vi "EnqueueCommand.vi"(8 "error in (no error)":errorcluster, 10 "element":T1, 11 "ResultProcessor in":refnum<class "ResultProcessor.lvclass">) -> (0 "error out":errorcluster, 3 "ResultProcessor out":refnum<class "ResultProcessor.lvclass">)   [LabVIEW 2015, in "ResultProcessor.lvclass"]
uses:
  ResultProcessor.lvclass
  CommandQueueDataType.ctl
  Report Information/Report Information.lvclass
  Result/Result.lvclass
  ResultProcessor.lvclass/ResultProcessor.ctl
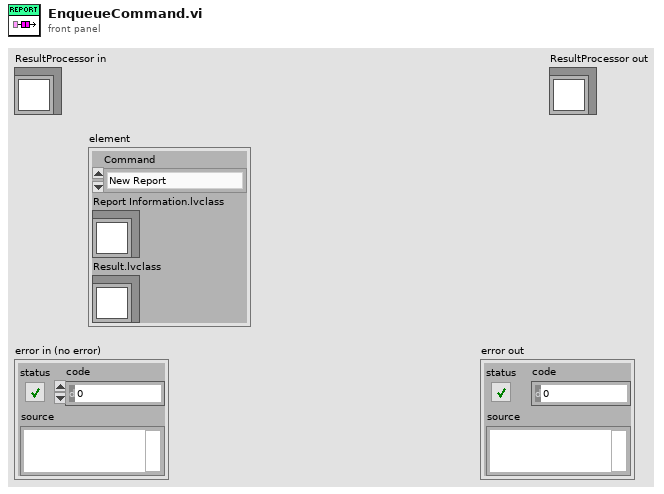
[diagram p1: front panel]
types:
  T1 = typedef "ResultProcessor.lvclass/CommandQueueDataType.ctl" = cluster{"Command":enum16{"New Report", "Add Result", "Publish Report", "Shutdown", "Add DUT Information", "Add Station Information", "Add Report Information", "Add Test Information"}, "Report Information.lvclass":refnum<class "Report Information.lvclass">, "Result.lvclass":refnum<class "Result.lvclass">}
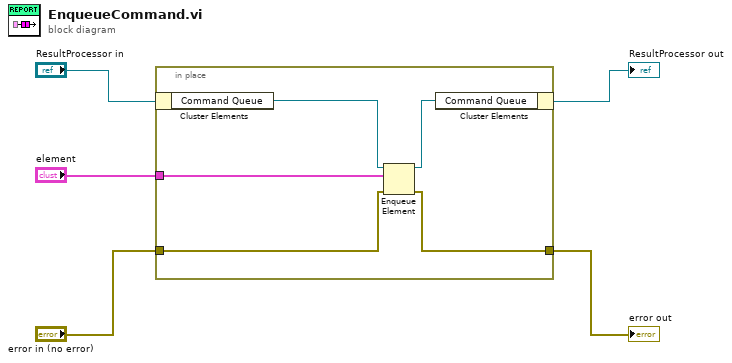
[diagram p0: block diagram]
diagram:
  n1 = in-place {
    in-place-border: "error in (no error)" -> [w8]
    in-place-border: [w7] -> w3
    in-place-border: "element" -> [w6]
    n2 = in-place-cluster #1("ResultProcessor in") -> ("Command Queue"=w10:refnum<queue>)
    n3 = Enqueue Element(queue=w10, element=w6, error in (no error)=w8) -> (queue out=w9:refnum<queue>, error out=w7:errorcluster)  [unwired: 1 in, 1 out]
    n4 = in-place-cluster #1("Command Queue"=w9) -> (→"ResultProcessor out":refnum<class "ResultProcessor.lvclass">)
  }
  "error out" <- w3
